vi "EngineStopped.vi"(10 "Engine Stopped Event Data":T1, 11 "Engine Event Interface in":refnum<class "EngineEventHandler-UserEvent.lvclass">) -> ()   [LabVIEW 2020, in "GLF.lvlib" / "EngineEventHandler-UserEvent.lvclass"]
uses:
  EngineEventHandler-UserEvent.lvclass
  EngineEventHandler-UserEvent.lvclass/EngineEventHandler-UserEvent.ctl
  EngineEventInterface/EngineStopped-EventData--cluster.ctl
  EngineEventInterface/EngineEventInterface.lvclass
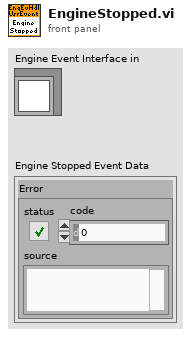
[diagram p1: front panel]
types:
  T1 = typedef "GLF.lvlib/EngineEventInterface.lvclass/EngineStopped-EventData--cluster.ctl" = cluster{"Error":errorcluster}
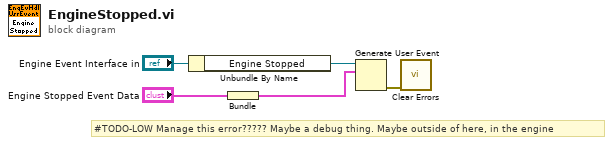
[diagram p0: block diagram]
diagram:
  # "#TODO-LOW Manage this error????? Maybe a debug thing. Maybe outside of here, in the engine"
  n1 = Unbundle By Name("Engine Event Interface in") -> ("Engine Stopped"=w4:refnum<user-event>)
  n2 = Bundle("Engine Stopped Event Data"="Engine Stopped Event Data") -> (w2:cluster{"Engine Stopped Event Data":T1})  [unwired: 1 in]
  n3 = Generate User Event(user event=w4, event data cluster=w2) -> (error out=w1:errorcluster)  [unwired: 2 in, 1 out]
  n4 = call <vilib>:"Clear Errors.vi"("error in (no error)"=w1) -> ()  [unwired: 5 in, 2 out]
